vi "Save Configuration.vi"(8 "error in":errorcluster, 11 "Theme Config in":refnum<class "Theme Config.lvclass">) -> (0 "error out":errorcluster, 3 "Theme Config out":refnum<class "Theme Config.lvclass">)   [LabVIEW 2021, in "Theme Config.lvclass"]
doc: "save the changed values of the configuration class\n\n<b>Code Developed By:</b> +\nDaniel Coons +\nTechnology Service Corporation +\nwww.tsc.com/atcs"
uses:
  Theme Config.lvclass
  C:/Program Files/National Instruments/LabVIEW 2026/vi.lib/JDP Science/JSONtext/Config Files/Config File.lvclass
  <vilib>/JDP Science/JSONtext/Config Files/Config File.lvclass/Config File.ctl
  <vilib>/JDP Science/JSONtext/Config Files/Config File.lvclass
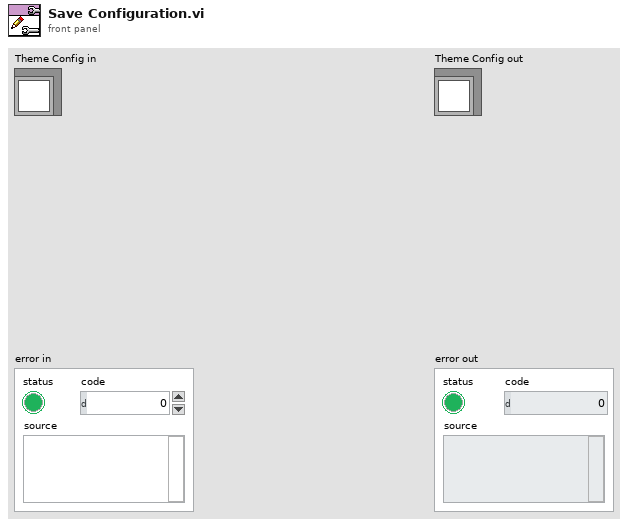
[diagram p1: front panel]
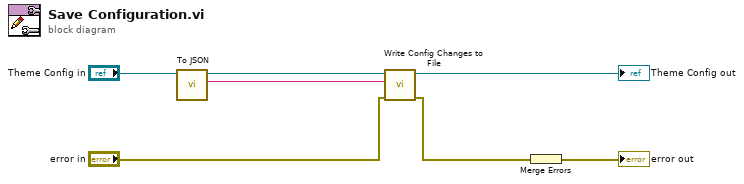
[diagram p0: block diagram]
diagram:
  n1 = call "To JSON.vi"("Theme Config in"="Theme Config in") -> ("JSON"=w3:string, "Theme Config out"=w5:refnum<class "Theme Config.lvclass">)  [unwired: 8 in, 1 out]
  n2 = call <vilib>:"Write Config Changes to File.vi"("error in (no error)"="error in", "New Config"=w3, "Config File in"=w5) -> ("error out"=w1:errorcluster, "Config File"=→"Theme Config out":refnum<class "Theme Config.lvclass">)  [unwired: 5 in, 2 out]
  n3 = Merge Errors(w1) -> (→"error out":errorcluster)
